vi "AIT 1553 - Create BC Sysdef Tree Acyclic Frames.vi"(8 "error in":errorcluster, 10 "Section Ptr":T1 format="%.0x", 11 "Acyclic_Frames":T2[](array[typedef])) -> (0 "error out":errorcluster, 2 "Section Ptr Out":T1 format="%.0x")   [LabVIEW 2013]
uses:
  <vilib>/NI Veristand/Custom Device API/Custom Device Item Ref.ctl
  Controls/1553_Acyclic_Frame.ctl
  <vilib>/NI Veristand/Custom Device API/Custom Device Channel.ctl
  <vilib>/NI Veristand/Custom Device API/Custom Device Channel Type.ctl
  <vilib>/NI Veristand/Custom Device API/Custom Device API.lvlib
  AIT 664 Custom Device.lvlib
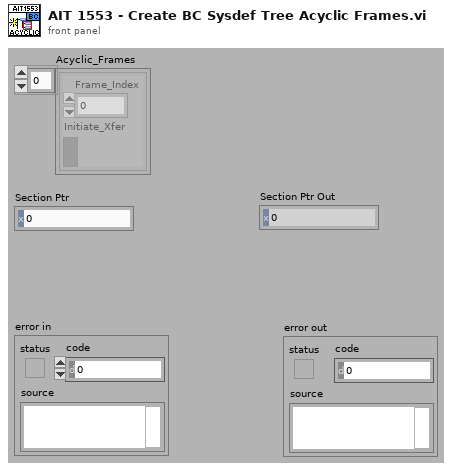
[diagram p1: front panel]
types:
  T1 = typedef "Custom Device API.lvlib/Custom Device Item Ref.ctl" = u64
  T2 = typedef "AIT 664 Custom Device.lvlib/1553_Acyclic_Frame.ctl" = cluster{"Frame_Index":u8, "Initiate_Xfer":bool}
  T3 = typedef "Custom Device API.lvlib/Custom Device Channel.ctl" = cluster{"Type":T4, "Units":string, "Default Value":dbl, "Faultable":bool, "Scalable":bool}
  T4 = typedef "Custom Device API.lvlib/Custom Device Channel Type.ctl" = enum16{"Input", "Output"}
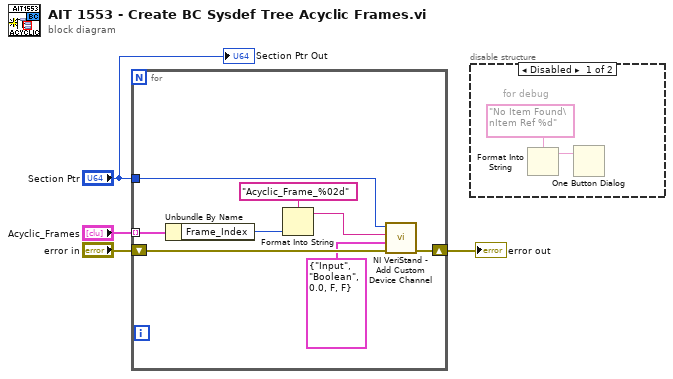
[diagram p0: block diagram]
diagram:
  n1 = for {
    shift-right: [w5] -> w4
    shift-left: "error in" -> [w12]
    tunnel: "Section Ptr" -> [w9]
    tunnel: "Acyclic_Frames" -> [w8] mode=indexing
    n2 = Unbundle By Name(w8) -> ("Frame_Index"=w7:u8)
    n3 = Format Into String(format string="Acyclic_Frame_%02d" ("Channel Name"), w7) -> (resulting string=w6:string)  [unwired: 2 in, 1 out]
    n4 = call <vilib>:"NI VeriStand - Add Custom Device Channel.vi"("error in (no error)"=w12, "Channel"=T3 {"Type"=enum."Input", "Units"="Boolean", "Default Value"=0.0, "Faultable"=FALSE, "Scalable"=FALSE}, "Channel Name"=w6, "Parent Ref in"=w9) -> ("error out"=w5:errorcluster)  [unwired: 4 in, 3 out]
  }
  "error out" <- w4
  n5 = disable-structure shown="Disabled" {
    frame Disabled {
      # "for debug"
      n6 = Format Into String(format string="No Item Found\nItem Ref %d" ("message")) -> (resulting string=w15:string, w13:T1)  [unwired: 2 in, 1 out]
      n7 = One Button Dialog(message=w15) -> (true=w16:bool)  [unwired: 1 in]
    }
    frame Enabled {
    }
  }
  "Section Ptr Out" <- "Section Ptr"
